vi "External Register Updated.vi"(4 "Register Value(s)":u16[](array[numeric]), 6 "String Value":string, 8 "error in (no error)":errorcluster, 9 "Value":dbl, 10 "Label":string, 11 "MB Slave in":refnum<class "iC7-AFE.lvclass">) -> (0 "error out":errorcluster, 2 "Debug Cluster":cluster{string, string, "Value":dbl}, 3 "MB Slave out":refnum<class "iC7-AFE.lvclass">)   [LabVIEW 2021, in "iC7-AFE.lvclass"]
uses:
  iC7-AFE.lvclass
  MB Slave Simulator Base/MB Slave Simulator Base.lvclass
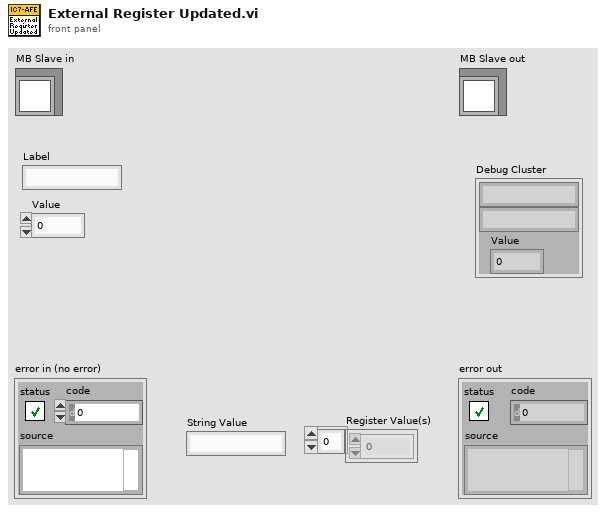
[diagram p1: front panel]
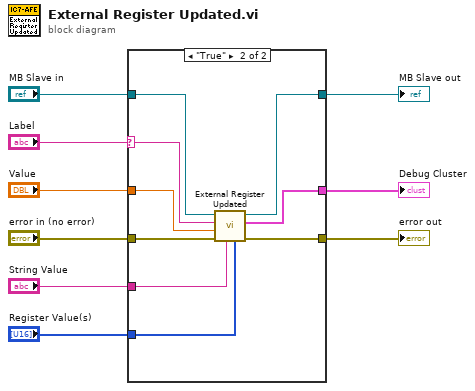
[diagram p0: block diagram]
diagram:
  n1 = case shown="\"True\"" "Label" {
    selector: "Label" -> [_ w13]
    tunnel: [w10 w20] -> w9
    tunnel: [_ w19] -> w8
    tunnel: [w11 w18] -> w7
    tunnel: "Register Value(s)" -> [_ w17]
    tunnel: "String Value" -> [_ w16]
    tunnel: "error in (no error)" -> [w10 w15]
    tunnel: "Value" -> [_ w14]
    tunnel: "MB Slave in" -> [w11 w12]
    frame "False", Default {
    }
    frame "True" {
      n2 = call-parent "External Register Updated.vi"("Register Value(s)"=w17, "String Value"=w16, "error in (no error)"=w15, "Value"=w14, "Label"=w13, "MB Slave in"=w12) -> ("error out"=w20:errorcluster, "Debug Cluster"=w19:cluster{string, string, "Value":dbl}, "MB Slave out"=w18:refnum<class "iC7-AFE.lvclass">)  [unwired: 3 in]
    }
  }
  "error out" <- w9
  "MB Slave out" <- w7
  "Debug Cluster" <- w8
